vi "COMMAND_GoToPosition.vi"(8 "error in (no error)":errorcluster, 10 "target  position":refnum<class "SpaceVector.lvclass">, 11 "StageDL090602SutterMP285 in":refnum<class "StageDL090602SutterMP285.lvclass">) -> (0 "error out":errorcluster, 3 "StageDL090602SutterMP285 out":refnum<class "StageDL090602SutterMP285.lvclass">)   [LabVIEW 2010, in "StageDL090602SutterMP285.lvclass"]
uses:
  StageDL090602SutterMP285.lvclass
  common/classes/SpaceVector/SpaceVector/SpaceVector.lvclass
  StageDL090602SutterMP285.lvclass/StageDL090602SutterMP285.ctl
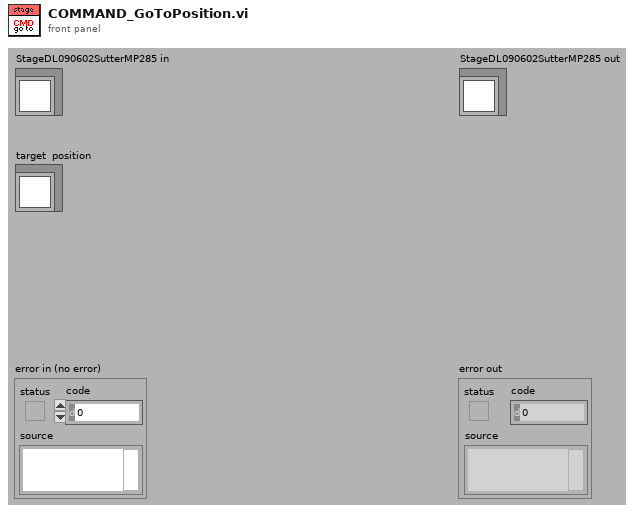
[diagram p1: front panel]
types:
  T1 = typedef "SpaceVector.lvclass/space_vector_array.ctl" = dbl[unit][]
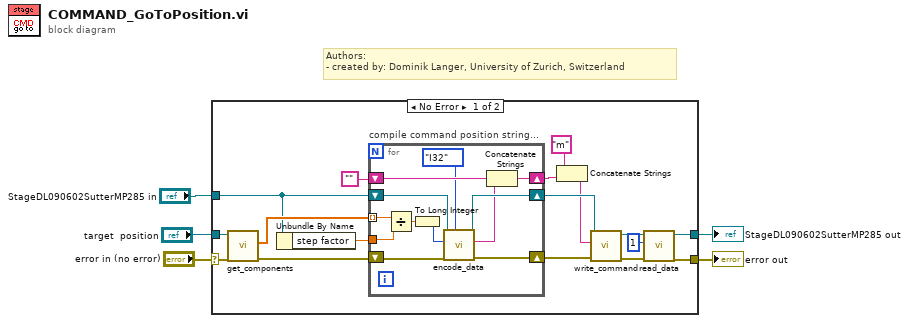
[diagram p0: block diagram]
diagram:
  # "Authors: \n- created by: Dominik Langer, University of Zurich, Switzerland"
  n1 = case shown="No Error" "error in (no error)" {
    selector: "error in (no error)" -> [w10 w36]
    tunnel: [w9 w36] -> w4
    tunnel: [w8 w35] -> w2
    tunnel: "StageDL090602SutterMP285 in" -> [w6 w35]
    tunnel: "target  position" -> [w11 _]
    frame No Error {
      n2 = call "get_components.vi"("error in (no error)"=w10, "SpaceVector in"=w11) -> ("error out"=w21:errorcluster, "x/y/z"=w22:T1)  [unwired: 8 out]
      n3 = Unbundle By Name(w6) -> ("step factor"=w7:dbl[unit])
      n4 = for "compile command position string..." {
        tunnel: w22 -> [w32] mode=indexing
        shift-right: [w30] -> w16
        shift-left: w6 -> [w24]
        shift-right: [w29] -> w20
        shift-left: w21 -> [w34]
        shift-right: [w27] -> w18
        shift-left: "" -> [w28]
        tunnel: w7 -> [w23]
        n5 = Divide(x=w32, y=w23) -> (x/y=w31:dbl)
        n6 = To Long Integer(number=w31) -> (32bit integer=w33:i32)
        n7 = call-dynamic "encode_data.vi"("data type"=enum16{"U16", "I32"}."I32", "error in (no error)"=w34, "data I32"=w33, "DL090602SutterMP285Stage in"=w24) -> ("error out"=w29:errorcluster, "encoded data"=w25:string, "DL090602SutterMP285Stage out"=w30:refnum<class "StageDL090602SutterMP285.lvclass">)  [unwired: 5 out]
        n8 = Concatenate Strings(w28, w25) -> (w27:string)
      }
      n9 = Concatenate Strings("m" ("string"), w18) -> (w12:string)
      n10 = call-dynamic "write_command.vi"("error in (no error)"=w20, "command (without terminating \"\\n\")"=w12, "DL090602SutterMP285Stage in"=w16) -> ("error out"=w15:errorcluster, "DL090602SutterMP285Stage out"=w14:refnum<class "StageDL090602SutterMP285.lvclass">)  [unwired: 7 out]
      n11 = call-dynamic "read_data.vi"("error in (no error)"=w15, "bytes to read"=u32 1, "DL090602SutterMP285Stage in"=w14) -> ("error out"=w9:errorcluster, "DL090602SutterMP285Stage out"=w8:refnum<class "StageDL090602SutterMP285.lvclass">)  [unwired: 7 out]
    }
    frame Error {
    }
  }
  "error out" <- w4
  "StageDL090602SutterMP285 out" <- w2
